vi "ServoHereToClearErrorDll.vi"(8 "error in":errorcluster, 9 "Stage":T1, 11 "DevRefIn":u32) -> (0 "error out":errorcluster, 2 "result string":string, 3 "DevRefOut":u32)   [LabVIEW 2020]
uses:
  StageSelector--Enum.ctl
  Galil/resources/gclib32/gclib32.lvlib
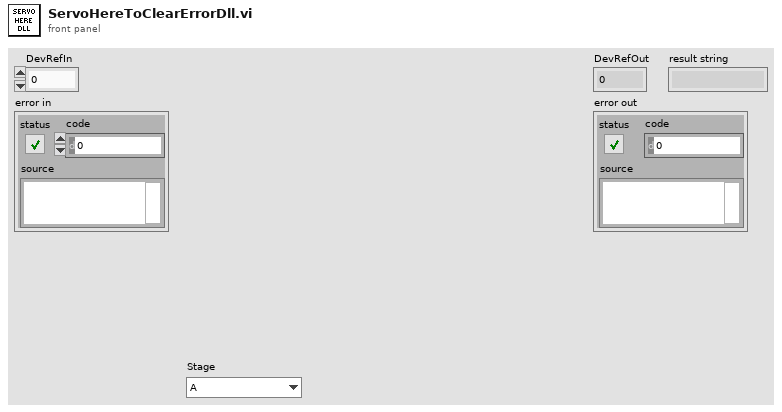
[diagram p1: front panel]
types:
  T1 = typedef "StageSelector--Enum.ctl" = enum16{"A", "B", "C", "D"}
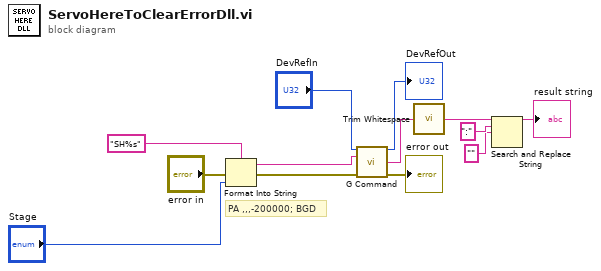
[diagram p0: block diagram]
diagram:
  # "PA ,,,-200000; BGD"
  n1 = Format Into String(format string="SH%s", error in="error in", "Stage") -> (resulting string=w4:string, error out=w7:errorcluster)  [unwired: 1 in]
  n2 = call "G Command.vi"("g"="DevRefIn", "command"=w4, "error in (no error)"=w7) -> ("g out"=→"DevRefOut":u32, "buffer out"=w5:string, "error out"=→"error out":errorcluster)  [unwired: 10 in]
  n3 = call <vilib>:"Trim Whitespace.vi"("string"=w5) -> ("trimmed string"=w12:string)  [unwired: 1 in]
  n4 = Search and Replace String(input string=w12, search string=":", replace string="" ("replace string (\"\")")) -> (result string=→"result string":string)  [unwired: 5 in, 3 out]
